vi "Validate Login.vi"(8 "error in":errorcluster, 9 "Password":string, 10 "UserName":string, 11 "connection reference":T1) -> (0 "error out":errorcluster, 2 "Level":string, 3 "Valid?":bool)   [LabVIEW 2018]
doc: "Checks validity of given user credentials."
uses:
  <vilib>/addons/database/Connection.llb/Conn ObjectReference.ctl
  <vilib>/addons/database/NI_Database_API.lvlib
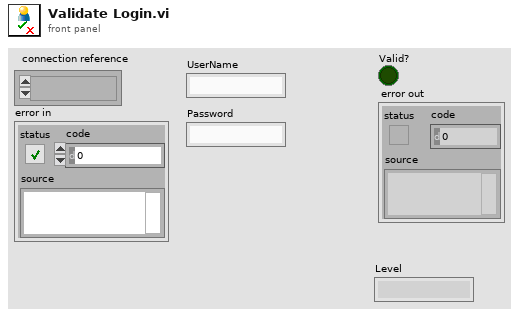
[diagram p1: front panel]
types:
  T1 = typedef "NI_Database_API.lvlib/Conn ObjectReference.ctl" = refnum<k1>
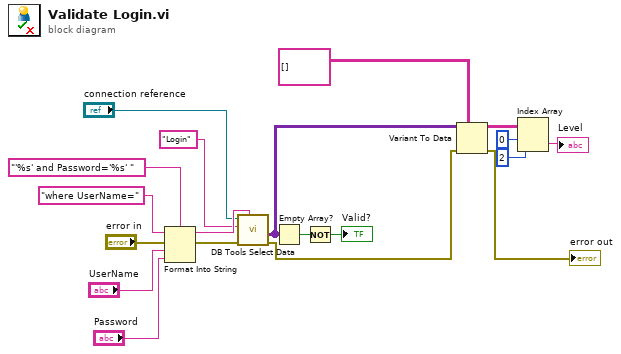
[diagram p0: block diagram]
diagram:
  n1 = Format Into String(format string="'%s' and Password='%s' ", initial string="where UserName=" ("condition"), error in="error in", "UserName", "Password") -> (resulting string=w17:string, error out=w15:errorcluster)
  n2 = call <vilib>:"DB Tools Select Data.vi"("condition"=w17, "error in (no error)"=w15, "table"="Login", "connection reference"="connection reference") -> ("error out"=w7:errorcluster, "data"=w9:variant[][])  [unwired: 2 in, 1 out]
  n3 = Empty Array?(array=w9) -> (empty?=w14:bool)
  n4 = Not(x=w14) -> (.not. x?=→"Valid?":bool)
  n5 = Variant To Data(error in=w7, type=string[][] [], Variant=w9) -> (data=w5:string[][], error out=→"error out":errorcluster)
  n6 = Index Array(array=w5, index (row)=0, index (col)=2 ("disabled index (col)")) -> (element=→"Level":string)
